vi "Set All SLSC Switch Properties.vi"(8 "error in":errorcluster, 10 "properties":T1, 11 "slsc switch custom device in":T2 format="%.0x") -> (0 "error out":errorcluster, 3 "slsc switch custom device out":T2 format="%.0x")   [LabVIEW 2020, in "SLSC Switch Scripting.lvlib"]
uses:
  SLSC Switch Scripting.lvlib
  <vilib>/NI VeriStand/Custom Device API/Custom Device Item Ref.ctl
  SLSC Switch All Properties.ctl
  <vilib>/NI VeriStand/Custom Device API/Custom Device API.lvlib
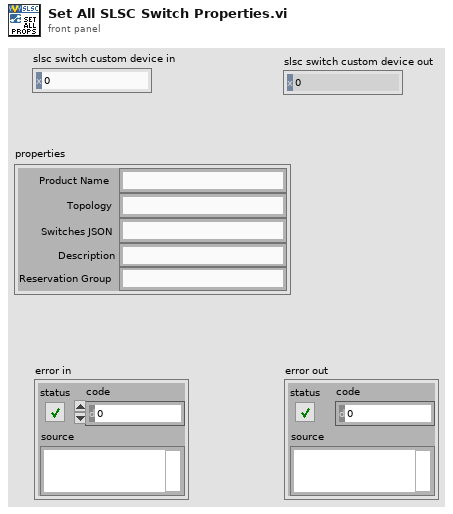
[diagram p1: front panel]
types:
  T1 = typedef "SLSC Switch Scripting.lvlib/SLSC Switch All Properties.ctl" = cluster{"Product Name":string, "Topology":string, "Switches JSON":string, "Description":string, "Reservation Group":string}
  T2 = typedef "Custom Device API.lvlib/Custom Device Item Ref.ctl" = u64
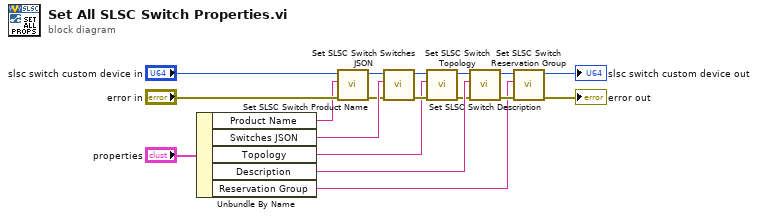
[diagram p0: block diagram]
diagram:
  n1 = Unbundle By Name("properties") -> ("Product Name"=w15:string, "Switches JSON"=w10:string, "Topology"=w9:string, "Description"=w13:string, "Reservation Group"=w1:string)
  n2 = call "Set SLSC Switch Product Name.vi"("error in"="error in", "product name"=w15, "slsc switch custom device in"="slsc switch custom device in") -> ("error out"=w5:errorcluster, "slsc switch custom device out"=w6:T2)  [unwired: 7 in]
  n3 = call "Set SLSC Switch Switches JSON.vi"("error in"=w5, "switches json"=w10, "slsc switch custom device in"=w6) -> ("error out"=w12:errorcluster, "slsc switch custom device out"=w8:T2)  [unwired: 7 in]
  n4 = call "Set SLSC Switch Topology.vi"("error in"=w12, "topology"=w9, "slsc switch custom device in"=w8) -> ("error out"=w11:errorcluster, "slsc switch custom device out"=w7:T2)  [unwired: 7 in]
  n5 = call "Set SLSC Switch Description.vi"("error in"=w11, "description"=w13, "slsc switch custom device in"=w7) -> ("error out"=w14:errorcluster, "slsc switch custom device out"=w3:T2)  [unwired: 7 in]
  n6 = call "Set SLSC Switch Reservation Group.vi"("error in"=w14, "reservation group"=w1, "slsc switch custom device in"=w3) -> ("error out"=→"error out":errorcluster, "slsc switch custom device out"=→"slsc switch custom device out":T2)  [unwired: 7 in]
